vi "Setup.vi"(5 "Protocol selection\n(appended)":T1 {"Mode" items=["Modbus-1", "3"]}, 7 "protocol selection ref":refnum<vi>, 8 "error in (no error)":errorcluster, 9 "search":bool, 10 "Comm master cluster in":T4={"Main event var"=refnum, "VIRef"=refnum, "Data path"=path "", "Reads"=0, "total number of UUT"=0, "FF refnum"={"Handle1"=0, "Handle2"=0}, "FF device id list"=[], "MODBUS resource name"="", "MODBUS Serial Parameters"={"Mode"=enum."RTU", "Default Slave Address"=0, "MODBUS timeout"=0, "Baud Rate"=0, "Parity"=0, "Flow Control"=0}, "Profibus resource name"="", "Profibus Communication ref.:"=0, "HART resource name"="", "HART long addresses (array)"=[], "Comm relay session"="", "Comm UI event"=refnum, "Write Interval (s)"=5.0, "DMM_QUEUE"=refnum, "POWER_QUEUE"=refnum, "\nTHERM_QUEUE"=refnum, "\nCOMM_QUEUE"=refnum, "TIMING_QUEUE"=refnum, "MAIN_QUEUE"=refnum, "Log path"=path ""} {"Write Interval (s)" min=0.1 max=1000.0 step=0.1}, 11 "Profibus in":refnum<class "Profibus.lvclass">) -> (0 "error out":errorcluster, 3 "Profibus out":refnum<class "Profibus.lvclass">)   [LabVIEW 2016, in "Profibus.lvclass"]
uses:
  Profibus.lvclass
  MASTER_OPC.ctl
  Typedef/event var.ctl
  Typedef/Comm ui action type.ctl
  Typedef/Comm_State_enum.ctl
  Typedef/state var.ctl
  Typedef/Array_of_Comm_mode_and_address_types.ctl
  Typedef/Comm_mode_and_address_type.ctl
  Typedef/Comm_mode_type_combo.ctl
  Typedef/Protocol_enum_type.ctl
  Profibus VISA Driver/DF PROFI II.llb/DFP2_Initialisation.ctl
  Profibus.lvclass/Profibus.ctl
  Protocol Class/Protocol.lvclass
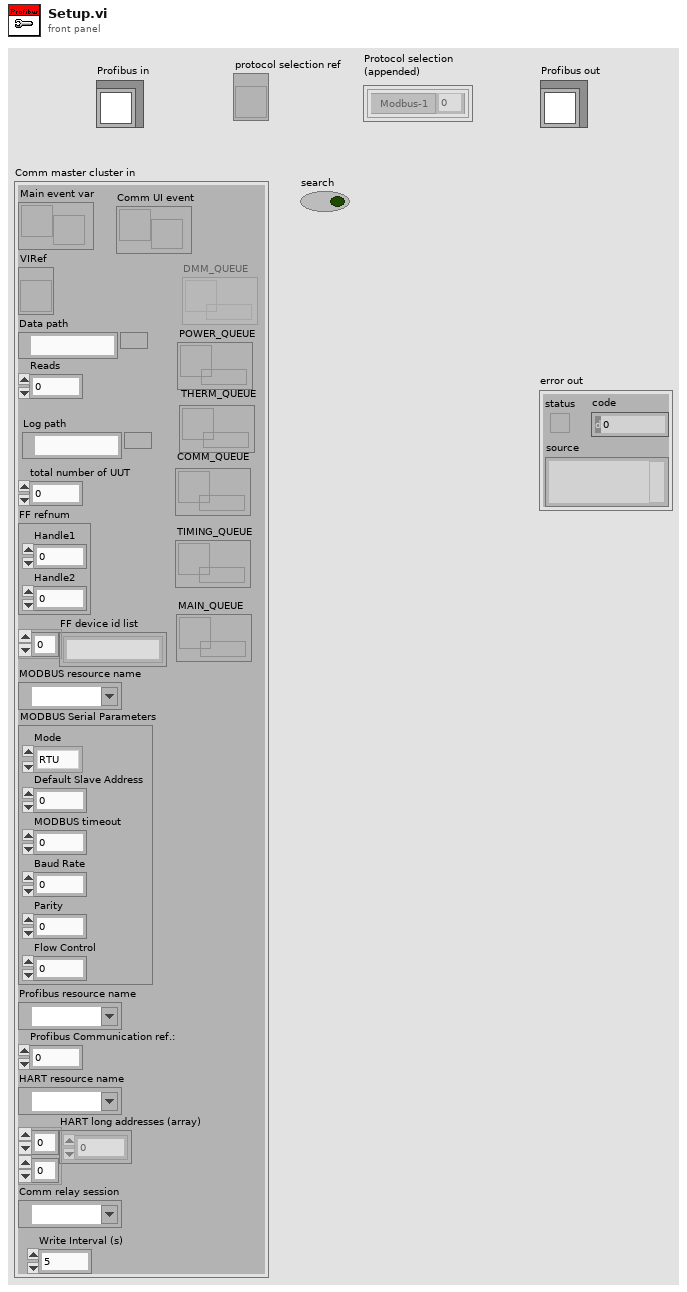
[diagram p1: front panel]
types:
  T1 = typedef "Array_of_Comm_mode_and_address_types.ctl" = T2[]
  T2 = typedef "Comm_mode_and_address_type.ctl" = cluster{"address":i32, "Mode":T3}
  T3 = typedef "Comm_mode_type_combo.ctl" = u16
  T4 = typedef "MASTER_OPC.ctl" = cluster{"Main event var":refnum<user-event>, "VIRef":refnum<vi>, "Data path":path, "Reads":i32, "total number of UUT":i32, "FF refnum":cluster{"Handle1":u32, "Handle2":u32}, "FF device id list":string[], "MODBUS resource name":refnum<visa-resource-name>, "MODBUS Serial Parameters":cluster{"Mode":enum16{"RTU", "ASCII"}, "Default Slave Address":u8, "MODBUS timeout":u32, "Baud Rate":u32, "Parity":u16, "Flow Control":u16}, "Profibus resource name":refnum<visa-resource-name>, "Profibus Communication ref.:":u8, "HART resource name":refnum<visa-resource-name>, "HART long addresses (array)":u8[][], "Comm relay session":refnum<k15>, "Comm UI event":refnum<user-event>, "Write Interval (s)":dbl, "DMM_QUEUE":refnum<queue>, "POWER_QUEUE":refnum<queue>, "\nTHERM_QUEUE":refnum<queue>, "\nCOMM_QUEUE":refnum<queue>, "TIMING_QUEUE":refnum<queue>, "MAIN_QUEUE":refnum<queue>, "Log path":path}
  T5 = typedef "Protocol_enum_type.ctl" = enum16{"None", "MODBUS", "HART", "Fieldbus", "Profibus DP", "Profibus PA", "DeviceNET", "USB"}
  T6 = enum16{"Connect whole bus", "Connect individual UUTs", "Connect none"}
  T7 = cluster{"Profibus-Addr.":i32, "Baud rate":i32, "CfgData":u8[]}
  T8 = typedef "DFP2_Initialisation.ctl" = enum32{"InitDFProfiIIAsDP-Master", "InitDFProfiIIAsDP-Slave", "Abort"}
  T9 = cluster{"Device address":i32, "Switch index":i32, "Communication ref.:":u8}
  T10 = cluster{"Device address":i32, "Switch index":i32, "Communication ref.:":u8}[]
  T11 = cluster{"Error":bool, "Status":i32, "Info":string}
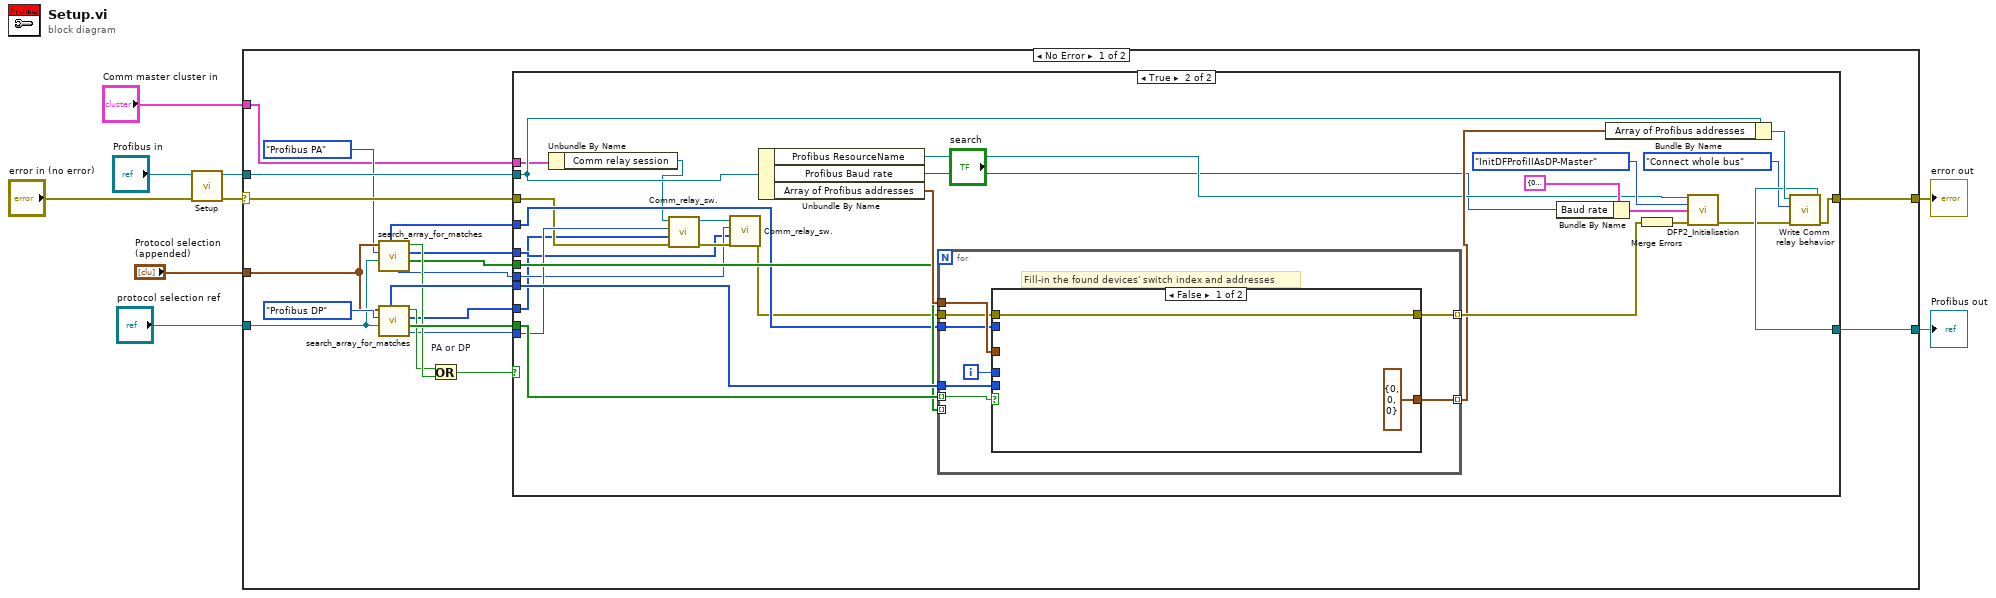
[diagram p0: block diagram]
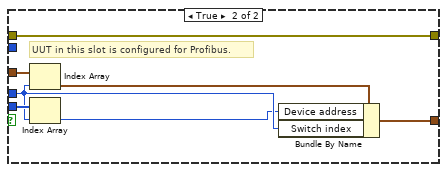
[diagram p3: hidden frame]
diagram:
  n1 = call-parent "Setup.vi"("error in (no error)"="error in (no error)", "Protocol in"="Profibus in") -> ("error out"=w7:errorcluster, "Protocol out"=w5:refnum<class "Profibus.lvclass">)  [unwired: 8 in]
  n2 = case shown="No Error" w7 {
    selector: w7 -> [w29 w78]
    tunnel: [w28 w78] -> w6
    tunnel: w5 -> [w27 w79]
    tunnel: [w25 w79] -> w4
    tunnel: "Comm master cluster in" -> [w14 _]
    tunnel: "Protocol selection\n(appended)" -> [w22 _]
    tunnel: "protocol selection ref" -> [w15 _]
    frame No Error {
      n3 = call "search_array_for_matches.vi"("protocol selection ref"=w15, "Protocol enum"=Protocol_enum_type."Profibus PA", "appended array"=w22) -> ("Array of exists"=w18:bool[], "array of indexes"=w11:i32[], "exists?"=w21:bool, "Switch Row"=w12:i32, "all addresses"=w17:i32[])  [unwired: 3 in, 1 out]
      n4 = call "search_array_for_matches.vi"("protocol selection ref"=w15, "Protocol enum"=Protocol_enum_type."Profibus DP", "appended array"=w22) -> ("Array of exists"=w24:bool[], "array of indexes"=w10:i32[], "exists?"=w20:bool, "Switch Row"=w13:i32, "all addresses"=w23:i32[])  [unwired: 3 in, 1 out]
      n5 = Or "PA or DP"(x=w20, y=w21) -> (x .or. y?=w19:bool)
      n6 = case shown="True" w19 {
        tunnel: w29 -> [w31 w44]
        tunnel: [w31 w32] -> w28
        tunnel: w27 -> [w30 w60]
        tunnel: w23 -> [_ w56]
        tunnel: [w30 w35] -> w25
        tunnel: w24 -> [_ w57]
        tunnel: w18 -> [_ w55]
        tunnel: w17 -> [_ w54]
        tunnel: w14 -> [_ w46]
        tunnel: w13 -> [_ w45]
        tunnel: w12 -> [_ w39]
        tunnel: w11 -> [_ w38]
        tunnel: w10 -> [_ w37]
        frame False {
        }
        frame True {
          n7 = Unbundle By Name(w46) -> ("Comm relay session"=w41:refnum<k15>)
          n8 = call "Comm_relay_sw..vi"("Error in"=w44, "Columns"=w37, "Row"=w45, "instrument handle in"=w41) -> ("error out"=w43:errorcluster, "instrument handle out"=w40:refnum<k15>)  [unwired: 6 in]
          n9 = call "Comm_relay_sw..vi"("Error in"=w43, "Columns"=w38, "Row"=w39, "instrument handle in"=w40) -> ("error out"=w42:errorcluster)  [unwired: 6 in, 1 out]
          n10 = Unbundle By Name(w60) -> ("Profibus ResourceName"=w49:refnum<visa-resource-name>, "Profibus Baud rate"=w48:i32, "Array of Profibus addresses"=w59:T10)
          n11 = for {
            tunnel: w59 -> [w68]
            tunnel: [w67] -> w53 mode=indexing
            tunnel: w42 -> [w66]
            tunnel: [w65] -> w58 mode=indexing
            tunnel: w57 -> [w64] mode=indexing
            tunnel: w56 -> [w62]
            tunnel: w55 -> [_] mode=indexing
            tunnel: w54 -> [w61]
            i -> [w63]
            # "Fill-in the found devices' switch index and addresses"
            n12 = case shown="False" w64 {
              tunnel: w68 -> [_ w72]
              tunnel: w62 -> [_ w77]
              tunnel: [T9 {"Device address"=0, "Switch index"=0, "Communication ref.:"=0} ("element") w73] -> w67
              tunnel: w66 -> [w70 w75]
              tunnel: [w70 w75] -> w65
              tunnel: w63 -> [_ w76]
              tunnel: w61 -> [_ _]
              frame False {
              }
              frame True {
                # "UUT in this slot is configured for Profibus."
                n13 = Index Array(array=w72, index=w76) -> (element=w71:T9)
                n14 = Index Array(array=w77, index=w76) -> (element=w74:i32)
                n15 = Bundle By Name(cluster=w71, "Device address"=w74, "Switch index"=w76) -> (w73:T9)
              }
            }
          }
          n16 = Bundle By Name(cluster=T7 {"Profibus-Addr."=0, "Baud rate"=10, "CfgData"=[]} ("DP-SlaveProperties:"), "Baud rate"=w48) -> (w52:T7)
          n17 = Bundle By Name(cluster=w60, "Array of Profibus addresses"=w53) -> (w36:refnum<class "Profibus.lvclass">)
          n18 = Merge Errors(w58) -> (w47:errorcluster)
          n19 = call "DFP2_Initialisation.vi"("DFP2ResourceName"=w49, "Mode"=DFP2_Initialisation."InitDFProfiIIAsDP-Master", "DP-SlaveProperties:"=w52, "ErrorIn:"=w47) -> ("ErrorOut:"=w33:T11)  [unwired: 9 in, 2 out]
          n20 = call-dynamic "Write Comm relay behavior.vi"("error in (no error)"=w33, "Comm relay behavior"=T6."Connect whole bus", "Protocol in"=w36) -> ("error out"=w32:errorcluster, "Protocol out"=w35:refnum<class "Profibus.lvclass">)  [unwired: 7 in]
        }
      }
    }
    frame Error {
    }
  }
  "error out" <- w6
  "Profibus out" <- w4
